vi "Get Calibration Table.vi"(8 "error in (no error)":errorcluster) -> (0 "error out":errorcluster, 1 "AO calibration data":string[][](array[string]), 3 "AI Calibration Table":string[][](array[string]))   [LabVIEW 2018]
uses:
  <vilib>/Utility/xml.llb/Read From XML File(string).vi
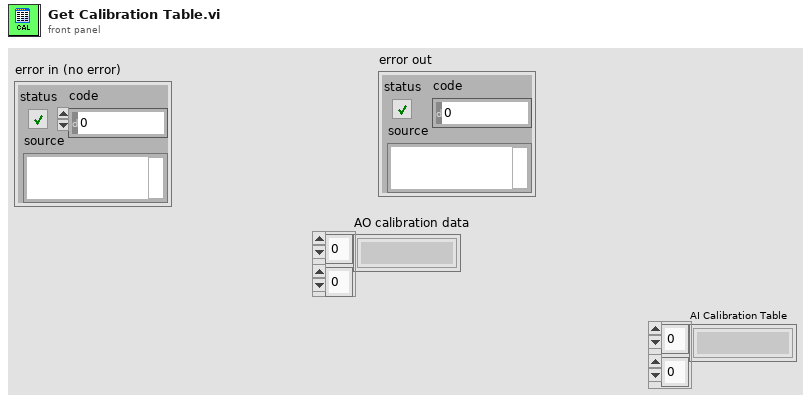
[diagram p1: front panel]
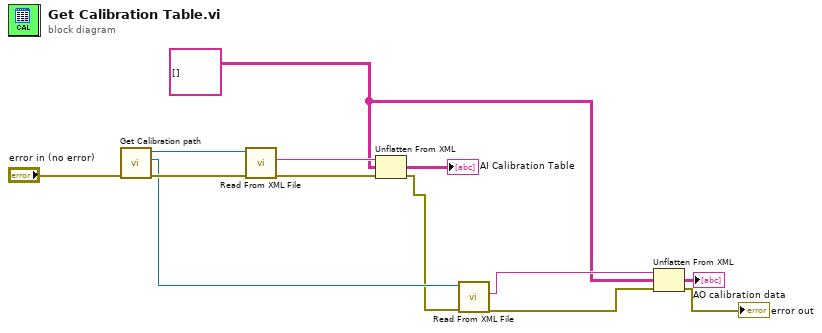
[diagram p0: block diagram]
diagram:
  w4 = string[][] []
  n1 = call "Get Calibration path.vi"("error in (no error)"="error in (no error)") -> ("error out"=w10:errorcluster, "AO Cal Path"=w7:path, "AI CAl Path"=w11:path)  [unwired: 8 in]
  n2 = call-poly <vilib>:"Read From XML File.vi"("error in (no error)"=w10, "XML File Path"=w11) -> ("error out"=w12:errorcluster, "XML Elements"=w13:string)  [unwired: 7 in, 1 out]
  n3 = Unflatten From XML(xml string=w13, type=w4, error in (no error)=w12) -> (value=→"AI Calibration Table":string[][], error out=w6:errorcluster)
  n4 = call-poly <vilib>:"Read From XML File.vi"("error in (no error)"=w6, "XML File Path"=w7) -> ("error out"=w3:errorcluster, "XML Elements"=w5:string)  [unwired: 7 in, 1 out]
  n5 = Unflatten From XML(xml string=w5, type=w4, error in (no error)=w3) -> (value=→"AO calibration data":string[][], error out=→"error out":errorcluster)
